vi "求阶乘（对数扩大范围）.vi"(1 "Num":i32=100) -> (0 "Fract（log）":dbl)   [LabVIEW 2012]
doc: "方法：\n\n利用公式直接计算阶乘时，由于数据大小变化剧烈，当n大于170时，很快会导致溢出。\n\n该VI采用对数的方式表示阶乘的结果，由于对数把乘法变成了加法，因此极大地扩展了计算范围。"
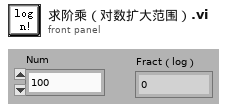
[diagram p1: front panel]
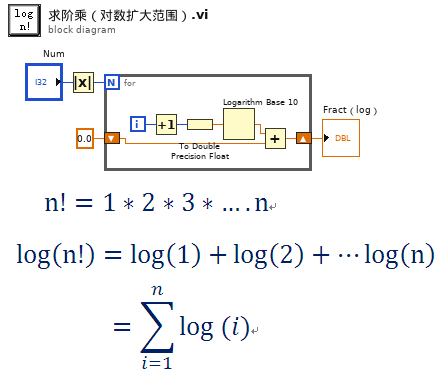
[diagram p0: block diagram]
diagram:
  n1 = Absolute Value(x="Num") -> (abs(x)=w3:i32)
  n2 = for {
    N: w3 -> [_]
    shift-right: [w6] -> w1
    shift-left: 0.0 -> [w5]
    i -> [w10]
    n3 = Increment(x=w10) -> (x+1=w9:i32)
    n4 = To Double Precision Float(number=w9) -> (double precision float=w7:dbl)
    n5 = Logarithm Base 10(1:w7) -> (0:w8:dbl)
    n6 = Add(x=w8, y=w5) -> (x+y=w6:dbl)
  }
  "Fract（log）" <- w1
